vi "Get Sections and Keys.vi"(7 "Section":string, 8 "error in":errorcluster, 11 "config-base in":refnum<class "config-base.lvclass">) -> (0 "error out":errorcluster, 1 "Keys":string[](array[string]), 2 "Sections":string[](array[string]), 3 "config-base out":refnum<class "config-base.lvclass">, 4 "Key Data Types":T1[](array[typedef]))   [LabVIEW 2022 SP3, in "hse-config.lvlib" / "config-base.lvclass"]
doc: "Returns all sub-sections, keys and the data types of the keys in a section.\n\n____\nHAMPEL SOFTWARE ENGINEERING v3.8.0 (2023-12-18 14:41)"
uses:
  config-base.lvclass
  <vilib>/Utility/Data Type/Type Definitions/Data Type.ctl
  config-base.lvclass/config-base.ctl
  <vilib>/Utility/Data Type/NI_Data Type.lvlib
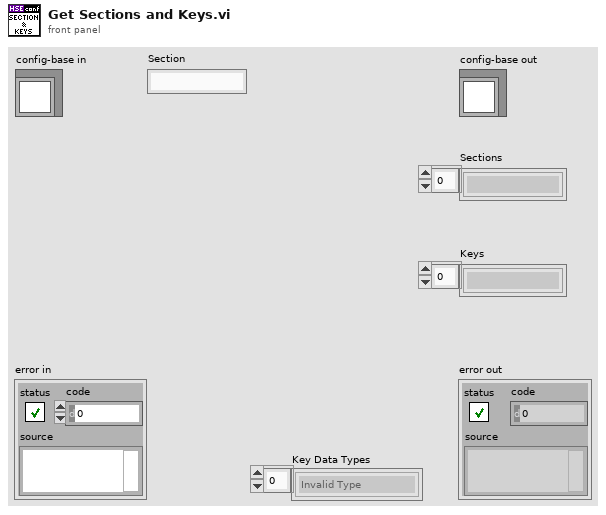
[diagram p1: front panel]
types:
  T1 = typedef "NI_Data Type.lvlib/Data Type.ctl" = enum8{"Invalid Type", "Void", "I8", "I16", "I32", "I64", "U8", "U16", "U32", "U64", "Single Float", "Double Float", "Extended Float", "Single Complex", "Double Complex", "Extended Complex", "Enum U8", "Enum U16", "Enum U32", "Enum U64", "Single Float With Unit", "Double Float With Unit", "Extended Float With Unit", "Single Complex with Unit", "Double Complex with Unit", "Extended Complex with Unit", "Boolean", "String", "Path", "Picture", "Tag", "Array", "Cluster", "Variant", "LV Variant", "Waveform", "Timestamp", "Digital Waveform", "Digital Data", "ExpressData", "Refnum", "External Data", "VI", "Poly VI", "LabVIEW Class Instance", "Fixed Point", "Set Collection", "Map Collection"}
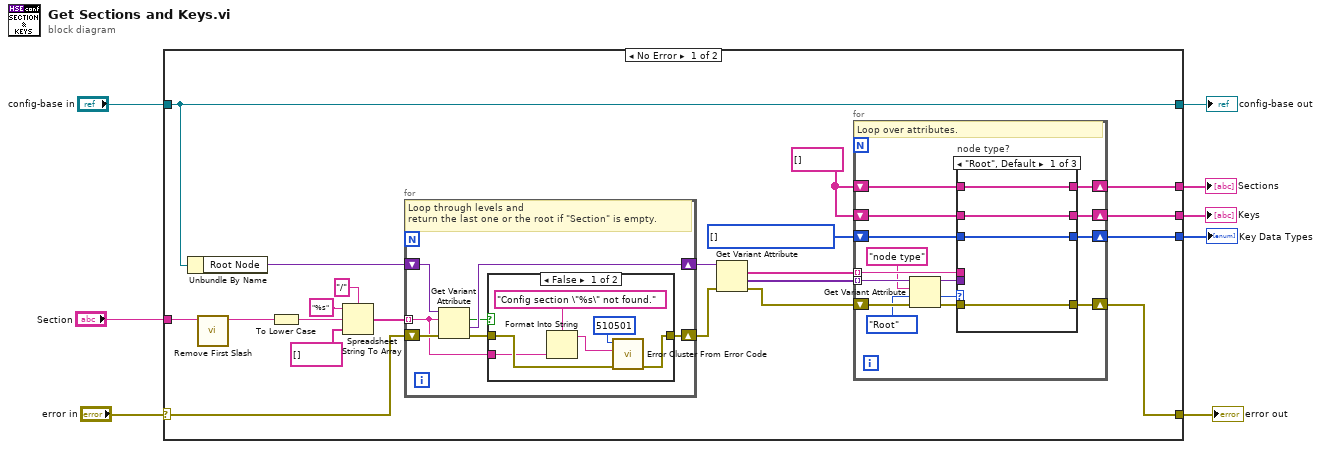
[diagram p0: block diagram]
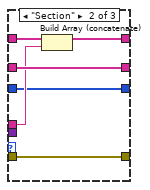
[diagram p3: hidden frame]
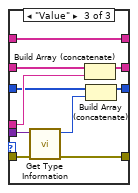
[diagram p4: hidden frame]
diagram:
  n1 = case shown="No Error" "error in" {
    selector: "error in" -> [w29 w80]
    tunnel: [w28 w79] -> w3
    tunnel: "config-base in" -> [w28 w79]
    tunnel: [w22 w80] -> w2
    tunnel: "Section" -> [w13 _]
    tunnel: [w21 _] -> w5
    tunnel: [w20 _] -> w4
    tunnel: [w10 _] -> w1
    frame No Error {
      w11 = T1[] [] items=["Invalid Type", "Void", "I8", "I16", "I32", "I64", "U8", "U16", "U32", "U64", "Single Float", "Double Float", "Extended Float", "Single Complex", "Double Complex", "Extended Complex", "Enum U8", "Enum U16", "Enum U32", "Enum U64", "Single Float With Unit", "Double Float With Unit", "Extended Float With Unit", "Single Complex with Unit", "Double Complex with Unit", "Extended Complex with Unit", "Boolean", "String", "Path", "Picture", "Tag", "Array", "Cluster", "Variant", "LV Variant", "Waveform", "Timestamp", "Digital Waveform", "Digital Data", "ExpressData", "Refnum", "External Data", "VI", "Poly VI", "LabVIEW Class Instance", "Fixed Point", "Set Collection", "Map Collection"]
      w23 = string[] []
      n2 = Unbundle By Name(w28) -> ("Root Node"=w27:variant)
      n3 = call "Remove First Slash.vi"("Section"=w13) -> ("result string"=w12:string)  [unwired: 10 in]
      n4 = To Lower Case(string=w12) -> (all lower case string=w9:string)
      n5 = Spreadsheet String To Array(delimiter (Tab)="/" ("Split Pattern"), format string="%s", spreadsheet string=w9, array type (2D Dbl)=string[] []) -> (array=w16:string[])
      n6 = for {
        shift-right: [w31] -> w14
        shift-left: w29 -> [w35]
        tunnel: w16 -> [w30] mode=indexing
        shift-right: [w34] -> w15
        shift-left: w27 -> [w36]
        # "Loop through levels and\nreturn the last one or the root if \"Section\" is empty."
        n7 = Get Variant Attribute(Variant=w36, name=w30, error in=w35) -> (found=w32:bool, value=w34:variant, error out=w33:errorcluster)  [unwired: 1 in, 1 out]
        n8 = case shown="False" w32 {
          tunnel: w33 -> [w42 w43]
          tunnel: [w41 w43] -> w31
          tunnel: w30 -> [w37 _]
          frame False {
            n9 = Format Into String(format string="Config section \"%s\" not found.", w37) -> (resulting string=w38:string)  [unwired: 2 in, 1 out]
            n10 = call <vilib>:"Error Cluster From Error Code.vi"("error in (no error)"=w42, "error message (\"\")"=w38, "error code (0)"=510501) -> ("error out"=w41:errorcluster)  [unwired: 6 in]
          }
          frame True {
          }
        }
      }
      n11 = Get Variant Attribute(Variant=w15, error in=w14) -> (names=w24:string[], values=w26:variant[], error out=w25:errorcluster)  [unwired: 2 in, 1 out]
      n12 = for {
        tunnel: w26 -> [w57] mode=indexing
        shift-right: [w44] -> w22
        shift-left: w25 -> [w55]
        tunnel: w24 -> [w58] mode=indexing
        shift-right: [w49] -> w21
        shift-left: w23 -> [w50]
        shift-right: [w48] -> w20
        shift-left: w23 -> [w51]
        shift-right: [w45] -> w10
        shift-left: w11 -> [w46]
        # "Loop over attributes."
        n13 = Get Variant Attribute(Variant=w57, name="node type", default value (empty Variant)=enum8{"Root", "Section", "Value"}."Root" ("Node Type"), error in=w55) -> (duplicate Variant=w52:variant, value=w53:enum8{"Root", "Section", "Value"}, error out=w47:errorcluster)  [unwired: 1 out]
        n14 = case "node type?" shown="\"Root\", Default" w53 {
          tunnel: w52 -> [_ _ w74]
          tunnel: w58 -> [_ w66 w75]
          tunnel: w51 -> [w61 w68 w77]
          tunnel: w50 -> [w62 w67 w78]
          tunnel: [w62 w65 w78] -> w49
          tunnel: [w61 w68 w76] -> w48
          tunnel: w47 -> [w59 w63 w73]
          tunnel: w46 -> [w60 w64 w72]
          tunnel: [w60 w64 w71] -> w45
          tunnel: [w59 w63 w69] -> w44
          frame "Root", Default {
          }
          frame "Section" {
            n15 = Build Array (concatenate)(w67, w66) -> (w65:string[])
          }
          frame "Value" {
            n16 = call <vilib>:"Get Type Information.vi"("error in (no error)"=w73, "variant"=w74) -> ("error out"=w69:errorcluster, "type"=w70:T1)  [unwired: 5 in, 3 out]
            n17 = Build Array (concatenate)(w77, w75) -> (w76:string[])
            n18 = Build Array (concatenate)(w72, w70) -> (w71:T1[])
          }
        }
      }
    }
    frame Error {
    }
  }
  "error out" <- w2
  "config-base out" <- w3
  "Sections" <- w5
  "Keys" <- w4
  "Key Data Types" <- w1
